vi "cmd.vi"(8 "错误输入":errorcluster caption="错误输入（无错误）", 9 "Cmd":string, 11 "连接ID":refnum<k5>) -> (0 "错误输出":errorcluster, 1 "Response":string, 3 "连接ID输出":refnum<k5>)   [LabVIEW 2017]
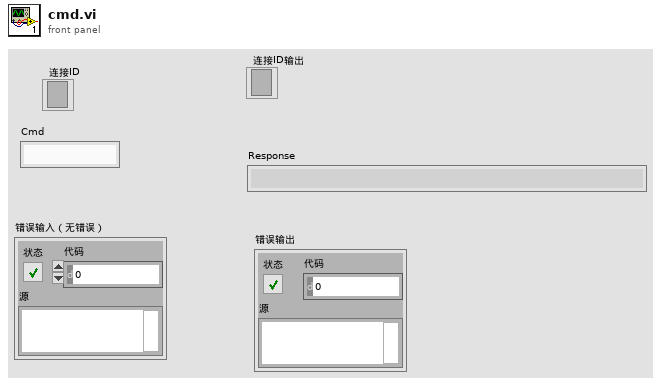
[diagram p1: front panel]
types:
  T1 = enum16{"Standard", "Buffered", "CRLF", "Immediate"}
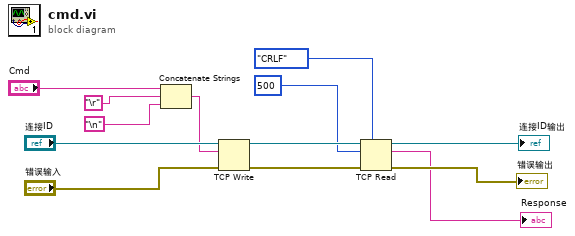
[diagram p0: block diagram]
diagram:
  n1 = Concatenate Strings("Cmd", "\r", "\n") -> (w1:string)
  n2 = TCP Write(connection ID="连接ID", data in=w1, error in (no error)="错误输入") -> (connection ID out=w13:refnum<k5>, error out=w12:errorcluster)  [unwired: 1 in, 1 out]
  n3 = TCP Read(connection ID=w13, bytes to read=500 ("读取的字节"), error in (no error)=w12, 7:T1."CRLF" ("模式（标准）")) -> (connection ID out=→"连接ID输出":refnum<k5>, data out=→"Response":string, error out=→"错误输出":errorcluster)  [unwired: 1 in]
